vi "IFilterPosition.vi"(0 "PRIORLib.IFilterIn":refnum<k7>, 1 "Wheel":i32=1) -> (2 "PRIORLib.IFilterOut":refnum<k7>, 3 "error out":errorcluster, 4 "Position":i16)   [LabVIEW 2016]
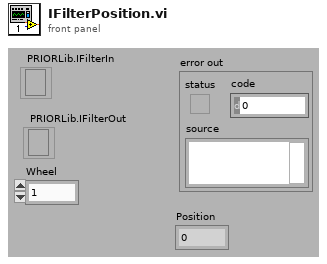
[diagram p1: front panel]
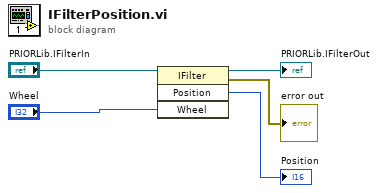
[diagram p0: block diagram]
diagram:
  n1 = invoke class="IFilter" method="Position"(reference="PRIORLib.IFilterIn", "Wheel"="Wheel") -> (reference out=→"PRIORLib.IFilterOut":refnum<k7>, error out=→"error out":errorcluster, "Position"=→"Position":i16)  [unwired: 2 in, 1 out]
